vi "example1.vi"() -> ()   [LabVIEW 2023]
uses:
  TCxxxx.lvlib
panel:
  out "temperature":dbl
  out "Read Buffer":string
  in  "VISA resource name":refnum<visa-resource-name>
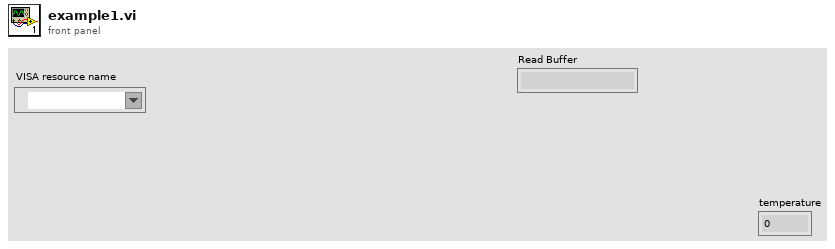
[diagram p1: front panel]
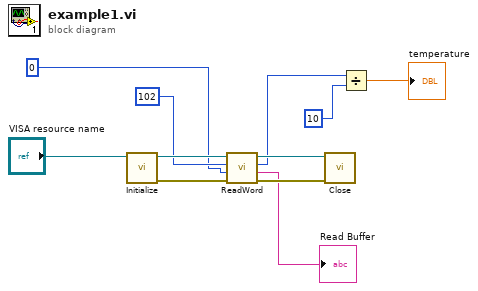
[diagram p0: block diagram]
diagram:
  n1 = call "Initialize.vi"("VISA resource name"="VISA resource name") -> ("error out"=w9:errorcluster, "VISA resource name out"=w11:refnum<visa-resource-name>)  [unwired: 9 in]
  n2 = call "ReadWord.vi"("error in (no error)"=w9, "Parameter [0 ... 65535]"=u16 0, "Befehl [0 ... 65535]"=u16 102, "VISA resource name"=w11) -> ("error out"=w8:errorcluster, "Read Buffer"=→"Read Buffer":string, "Regler Rückgabewert [0 ... 65535]"=w3:u16, "VISA resource name out"=w10:refnum<visa-resource-name>)  [unwired: 4 in]
  n3 = call "Close.vi"("error in (no error)"=w8, "VISA resource name"=w10) -> ()  [unwired: 9 in, 1 out]
  n4 = Divide(x=w3, y=u16 10) -> (x/y=→"temperature":dbl)
